vi "Adept - Stream To Register.vi"() -> ()   [LabVIEW 2011]
uses:
  vi.lib/LabVIEW Hacker/Adept/Private/Type Defs/Adept Device Ctl.xctl
  vi.lib/LabVIEW Hacker/Adept/Public/Write 1 Register.vi
  vi.lib/LabVIEW Hacker/Adept/LVH-Adept.lvlib
panel:
  in  "milliseconds to wait":u32
  in  "Stop Button":bool
  in  "Register Address":u8
  in  "Adept Device":u16(xcontrol)
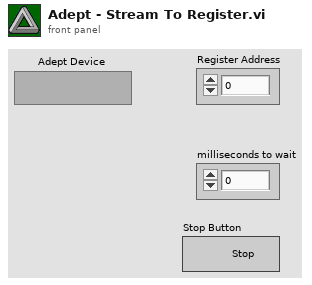
[diagram p1: front panel]
types:
  T1 = typedef "LVH-Adept.lvlib/Device Config.ctl" = cluster{"Num Devices":i32, "Device Names":string[], "Device Index":u16, "Device Handle":u32, "Status":T2}
  T2 = typedef "LVH-Adept.lvlib/Status.ctl" = cluster{"DEPP":bool, "DSTM":bool, "DJTG":bool}
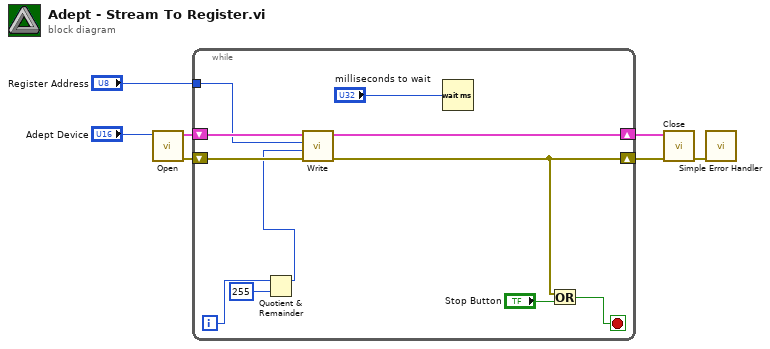
[diagram p0: block diagram]
diagram:
  n1 = call "Open.vi"("Adept Device"="Adept Device") -> ("Error Out"=w6:errorcluster, "Adept Config"=w7:T1)  [unwired: 9 in]
  n2 = while {
    tunnel: "Register Address" -> [w16]
    shift-right: [w13] -> w1
    shift-left: w6 -> [w17]
    shift-right: [w15] -> w2
    shift-left: w7 -> [w18]
    i -> [w11]
    stop <- w14 stop-if-true
    n3 = Quotient & Remainder(x=w11, y=255) -> (x-y*floor(x/y)=w9:i32)  [unwired: 1 out]
    n4 = call-poly "Write.vi"("Error In"=w17, "Data"=w9, "Register Address"=w16, "Adept Config"=w18) -> ("Error Out"=w13:errorcluster, "Adept Config"=w15:T1)  [unwired: 6 in]
    n5 = Wait (ms)(milliseconds to wait="milliseconds to wait") -> ()  [unwired: 1 out]
    n6 = Or(x=w13, y="Stop Button") -> (x .or. y?=w14:bool)
  }
  n7 = call "Close.vi"("Error In"=w1, "Adept Config"=w2) -> ("Error Out"=w5:errorcluster)  [unwired: 9 in]
  n8 = call <vilib>:"Simple Error Handler.vi"("error in (no error)"=w5) -> ()  [unwired: 4 in, 5 out]
